vi "verify parameter in list.vi"(8 "error in (no error)":errorcluster, 9 "value":u16, 10 "list of values":u16[](array[numeric]), 11 "parameter name":string) -> (0 "error out":errorcluster, 2 "verific error":errorcluster)   [LabVIEW 2018]
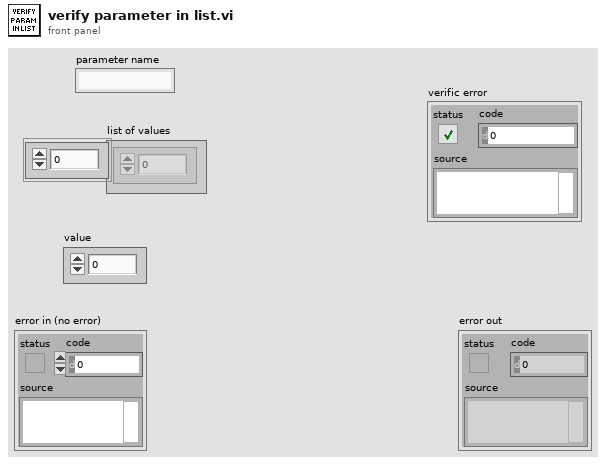
[diagram p1: front panel]
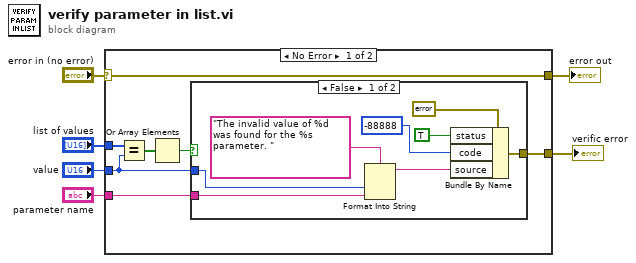
[diagram p0: block diagram]
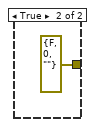
[diagram p2: hidden frame]
diagram:
  n1 = case shown="No Error" "error in (no error)" {
    selector: "error in (no error)" -> [w8 w23]
    tunnel: [w8 w23] -> w5
    tunnel: "list of values" -> [w13 _]
    tunnel: "value" -> [w9 _]
    tunnel: "parameter name" -> [w10 _]
    tunnel: [w7 _] -> w1
    frame No Error {
      n2 = Equal?(x=w13, y=w9) -> (x = y?=w12:bool[])
      n3 = Or Array Elements(Boolean array=w12) -> (logical OR=w11:bool)
      n4 = case shown="False" w11 {
        tunnel: w10 -> [w17 _]
        tunnel: w9 -> [w15 _]
        tunnel: [w14 errorcluster {"status"=FALSE, "code"=0, "source"=""} ("error constant")] -> w7
        frame False {
          n5 = Format Into String(format string="The invalid value of %d was found for the %s parameter. " ("source"), w15, w17) -> (resulting string=w16:string)  [unwired: 2 in, 1 out]
          n6 = Bundle By Name(cluster=errorcluster {"status"=FALSE, "code"=0, "source"=""} ("error constant"), "status"=TRUE, "code"=-88888, "source"=w16) -> (w14:errorcluster)
        }
        frame True {
        }
      }
    }
    frame Error {
    }
  }
  "error out" <- w5
  "verific error" <- w1
